vi "InitialiseLCD1602.vi"(5 "Address":u8=62 format="%.0x", 7 "Bus":u8, 8 "error in (no error)":errorcluster, 10 "I2C Options":T1={"Baud"=400000, "SCL GPIO"=10, "SDA GPIO"=9}, 11 "Port":refnum<visa-resource-name>="COM5") -> (0 "error out":errorcluster={"status"=FALSE, "code"=1073676294, "source"="VISA Read in CTI-Visa.lvlib:Read Response.vi->CTI-Visa.lvlib:Read Identity.vi->TestLCD.vi"}, 3 "VISA resource name":refnum<visa-resource-name>)   [LabVIEW 2024]
uses:
  Driver/Public/I2C Options.ctl
  Driver/Public/Digital Pull Direction.ctl
  7af1f806-0ba7-455a-9c2f-bbd77f8ada64.vi
  8ef2f78a-7123-4114-9f1a-89a7b321d551.vi
  Driver/CTIPicoVISA.lvlib
panel:
  # "Input"
  # "Output"
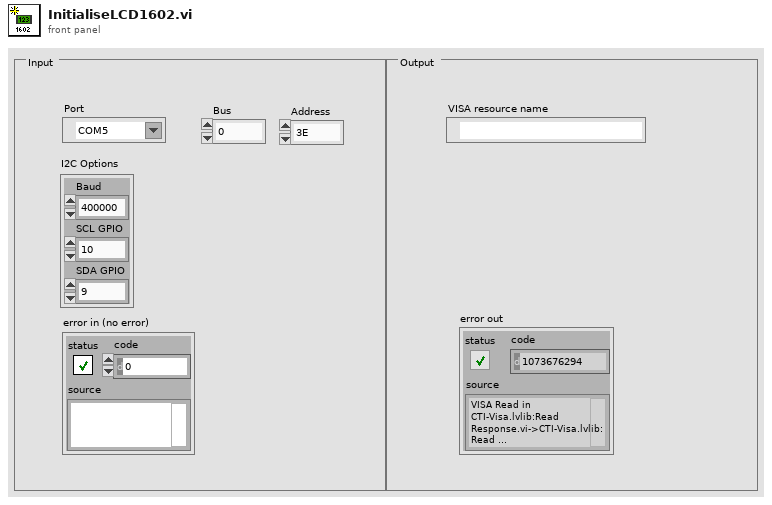
[diagram p1: front panel]
types:
  T1 = typedef "CTIPicoVISA.lvlib/I2C Options.ctl" = cluster{"Baud":u32, "SCL GPIO":i32, "SDA GPIO":i32}
  T2 = typedef "CTIPicoVISA.lvlib/Digital Pull Direction.ctl" = enum16{"None", "Up", "Down", "Both"}
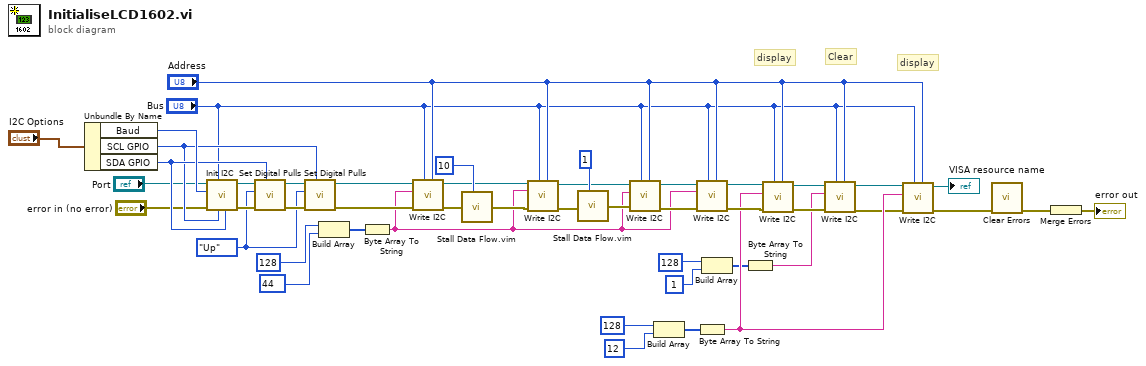
[diagram p0: block diagram]
diagram:
  w38 = Digital_Pull_Direction."Up" ("Pull")
  # "display"
  # "Clear"
  # "display"
  n1 = Unbundle By Name("I2C Options") -> ("Baud"=w45:u32, "SCL GPIO"=w39:i32, "SDA GPIO"=w42:i32)
  n2 = call "Init I2C.vi"("SDA GPIO"=w42, "SCL GPIO"=w39, "Bus"="Bus", "error in (no error)"="error in (no error)", "Baud"=w45, "VISA resource name in"="Port") -> ("error out"=w44:errorcluster, "VISA resource name"=w43:refnum<visa-resource-name>)  [unwired: 4 in]
  n3 = call "Set Digital Pulls.vi"("GPIO"=w42, "error in (no error)"=w44, "Pull"=w38, "VISA resource name in"=w43) -> ("error out"=w41:errorcluster, "VISA resource name"=w40:refnum<visa-resource-name>)  [unwired: 6 in]
  n4 = call "Set Digital Pulls.vi"("GPIO"=w39, "error in (no error)"=w41, "Pull"=w38, "VISA resource name in"=w40) -> ("error out"=w37:errorcluster, "VISA resource name"=w36:refnum<visa-resource-name>)  [unwired: 6 in]
  n5 = Build Array(u8 128 ("Value"), u8 44 ("Value")) -> (w35:u8[])
  n6 = Byte Array To String(unsigned byte array=w35) -> (string=w23:string)
  n7 = call "Write I2C.vi"("Address"="Address", "Bus"="Bus", "error in (no error)"=w37, "Data"=w23, "VISA resource name in"=w36) -> ("error out"=w34:errorcluster, "VISA resource name"=w30:refnum<visa-resource-name>)  [unwired: 5 in]
  n8 = call "Stall Data Flow.vim"("value in"=w34, "milliseconds to wait"=u32 10) -> ("value out"=w31:errorcluster)  [unwired: 1 out]
  n9 = call "Write I2C.vi"("Address"="Address", "Bus"="Bus", "error in (no error)"=w31, "Data"=w23, "VISA resource name in"=w30) -> ("error out"=w29:errorcluster, "VISA resource name"=w26:refnum<visa-resource-name>)  [unwired: 5 in]
  n10 = call "Stall Data Flow.vim"("value in"=w29, "milliseconds to wait"=u32 1) -> ("value out"=w27:errorcluster)  [unwired: 1 out]
  n11 = call "Write I2C.vi"("Address"="Address", "Bus"="Bus", "error in (no error)"=w27, "Data"=w23, "VISA resource name in"=w26) -> ("error out"=w25:errorcluster, "VISA resource name"=w24:refnum<visa-resource-name>)  [unwired: 5 in]
  n12 = Build Array(u8 128 ("Value"), u8 12 ("Value")) -> (w20:u8[])
  n13 = call "Write I2C.vi"("Address"="Address", "Bus"="Bus", "error in (no error)"=w25, "Data"=w23, "VISA resource name in"=w24) -> ("error out"=w22:errorcluster, "VISA resource name"=w21:refnum<visa-resource-name>)  [unwired: 5 in]
  n14 = Byte Array To String(unsigned byte array=w20) -> (string=w18:string)
  n15 = Build Array(u8 128 ("Value"), u8 1 ("Value")) -> (w12:u8[])
  n16 = Byte Array To String(unsigned byte array=w12) -> (string=w11:string)
  n17 = call "Write I2C.vi"("Address"="Address", "Bus"="Bus", "error in (no error)"=w22, "Data"=w18, "VISA resource name in"=w21) -> ("error out"=w16:errorcluster, "VISA resource name"=w14:refnum<visa-resource-name>)  [unwired: 5 in]
  n18 = call "Write I2C.vi"("Address"="Address", "Bus"="Bus", "error in (no error)"=w16, "Data"=w11, "VISA resource name in"=w14) -> ("error out"=w17:errorcluster, "VISA resource name"=w15:refnum<visa-resource-name>)  [unwired: 5 in]
  n19 = call "Write I2C.vi"("Address"="Address", "Bus"="Bus", "error in (no error)"=w17, "Data"=w18, "VISA resource name in"=w15) -> ("error out"=w3:errorcluster, "VISA resource name"=→"VISA resource name":refnum<visa-resource-name>)  [unwired: 5 in]
  n20 = call <vilib>:"Clear Errors.vi"("error in (no error)"=w3) -> ("error out"=w46:errorcluster)  [unwired: 5 in, 1 out]
  n21 = Merge Errors(w46) -> (→"error out":errorcluster)
